vi "API_InvokePPP_Python.vi"(6 "Timeout (ms)":u32, 7 "Wait (F)":bool, 8 "error in (no error)":errorcluster, 10 "PPP_parameters":T1={"product"="", "printer"="", "printhead"=enum."1", "material"="", "weight"=0.0, "density"=0.0, "overprint"=0.0, "print_wt_multiplier"=0.0, "num_of_drops"=0, "gs_source"="", "gs_val_file"=path "", "zone_compensation"=FALSE, "zone_comp_file"=path "", "bitmap"=path "", "save_gs_img"=FALSE, "dithered_save_path"=path "", "gs_save_path"=path "", "rotation"=FALSE, "driver"="", "server"="", "database"="", "user"="", "password"=""}, 11 "DLP2 in":refnum<class "DLP2.lvclass">) -> (0 "error out":errorcluster, 3 "DLP2 out":refnum<class "DLP2.lvclass">)   [LabVIEW 2022 SP3, in "DLP2.lvclass"]
doc: "Developed by Kevin Thompson\nkevin@thompsonengineering.net\n\nCopyright 2018\nThompson Engineering, LLC"
uses:
  DLP2.lvclass
  DataTypes/PPP_Python--cluster.ctl
  TopLevel/Typedefs/PrinterHeads--Enum.ctl
  DataTypes/AsynCmd_Temp01--enum.ctl
  DLP2.lvclass/DLP2.ctl
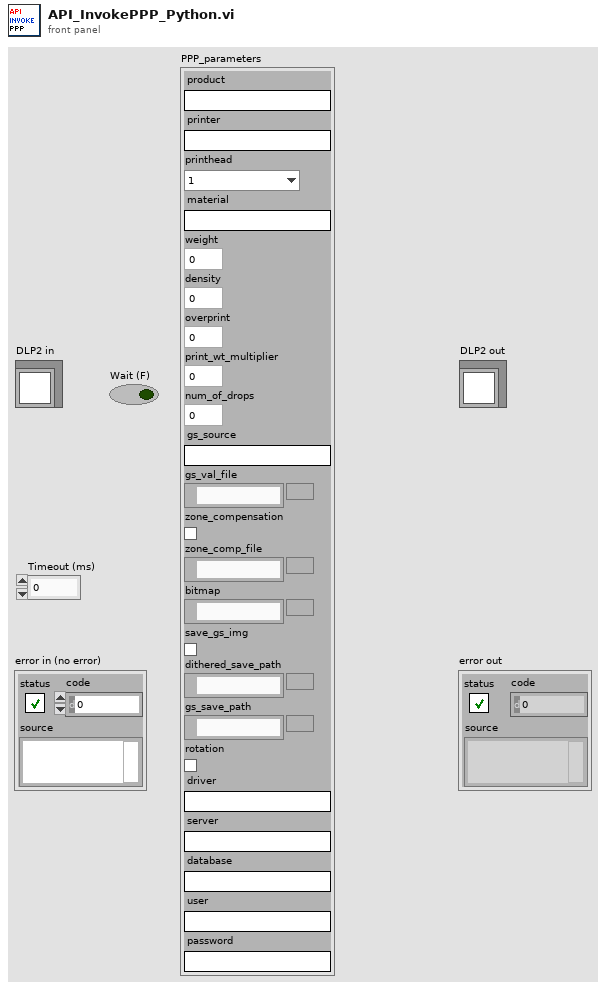
[diagram p1: front panel]
types:
  T1 = typedef "PPP_Python--cluster.ctl" = cluster{"product":string, "printer":string, "printhead":T2, "material":string, "weight":dbl, "density":dbl, "overprint":dbl, "print_wt_multiplier":dbl, "num_of_drops":i32, "gs_source":string, "gs_val_file":path, "zone_compensation":bool, "zone_comp_file":path, "bitmap":path, "save_gs_img":bool, "dithered_save_path":path, "gs_save_path":path, "rotation":bool, "driver":string, "server":string, "database":string, "user":string, "password":string}
  T2 = typedef "PrinterHeads--Enum.ctl" = enum16{"-1", "1", "2", "3", "4", "5", "6"}
  T3 = typedef "DLP2.lvclass/AsynCmd_Temp01--enum.ctl" = enum16{"LoadTiffImage", "SeperateLayersPython", "InvokePPP"}
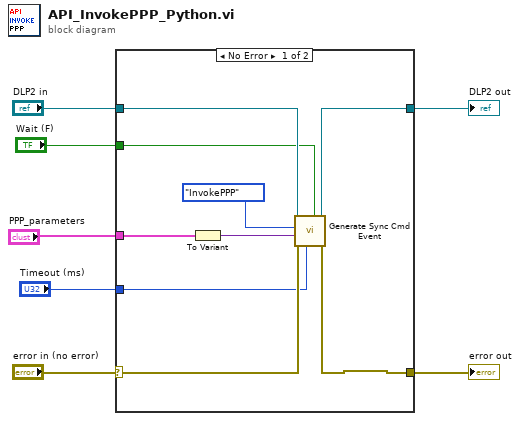
[diagram p0: block diagram]
diagram:
  n1 = case shown="No Error" "error in (no error)" {
    selector: "error in (no error)" -> [w14 w18]
    tunnel: [w8 w18] -> w6
    tunnel: [w15 w17] -> w4
    tunnel: "DLP2 in" -> [w16 w17]
    tunnel: "PPP_parameters" -> [w12 _]
    tunnel: "Wait (F)" -> [w10 _]
    tunnel: "Timeout (ms)" -> [w9 _]
    frame No Error {
      n2 = To Variant(anything=w12) -> (Variant=w11:variant)
      n3 = call "Generate Sync Cmd Event.vi"("Wait (F)"=w10, "Timeout (ms)"=w9, "error in (no error)"=w14, "vData"=w11, "AsyncCmd"=AsynCmd_Temp01--enum."InvokePPP", "DLP2 in"=w16) -> ("error out"=w8:errorcluster, "DLP2 out"=w15:refnum<class "DLP2.lvclass">)  [unwired: 3 in, 1 out]
    }
    frame Error {
    }
  }
  "error out" <- w6
  "DLP2 out" <- w4
